vi "Sync Time.vi"(0 "FPGA Timekeeper time (ns)":u64, 1 "time reference time (ns)":u64) -> ()   [LabVIEW 2015, in "FPGA Timekeeper.lvlib"]
doc: "Synchronizes the FPGA Timekeeper to a Time Reference (i.e. GPS, RT,...). To synchronize the FPGA Timekeeper to a Time Reference, call this VI periodically with the time of the Time Reference and the correlating time of the FPGA Timekeeper."
uses:
  FPGA Timekeeper.lvlib
  private/sync time event (g).vi
  <vilib>/rvi/Emulation/niFpgaSctlEmulationGetInTimedLoop.vi
  private/timereference time (g).vi
  <vilib>/rvi/Emulation/niFpgaProcessEmulError.vi
  private/timereference timestamp (g).vi
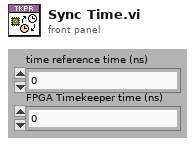
[diagram p1: front panel]
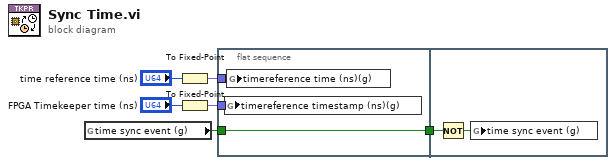
[diagram p0: block diagram]
diagram:
  n1 = global read "sync time event (g).vi" "time sync event (g)"() -> (w2:bool)
  n2 = To Fixed-Point(number="time reference time (ns)") -> (fixed-point=w4:fxp<+,64,64>)  [unwired: 1 in]
  n3 = To Fixed-Point(number="FPGA Timekeeper time (ns)") -> (fixed-point=w3:fxp<+,64,64>)  [unwired: 1 in]
  n4 = flat-sequence {
    tunnel: w3 -> [w8]
    tunnel: w4 -> [w9]
    tunnel: w2 -> [w7]
    tunnel: [w7] -> w1
    tunnel: w1 -> [w11]
    frame #0 {
      n5 = global write "timereference timestamp (g).vi" "timereference timestamp (ns)(g)"(w8) -> ()
      n6 = global write "timereference time (g).vi" "timereference time (ns)(g)"(w9) -> ()
    }
    frame #1 {
      n7 = Not(x=w11) -> (.not. x?=w10:bool)
      n8 = global write "sync time event (g).vi" "time sync event (g)"(w10) -> ()
    }
  }
